vi "Jeremy Example.vi"() -> ()   [LabVIEW 2016]
panel:
  in  "Path":path
  out "Waveform Graph 2":dbl[](graph)
  out "Time Stamp":timestamp
  out "Waveform Graph":dbl[](graph)
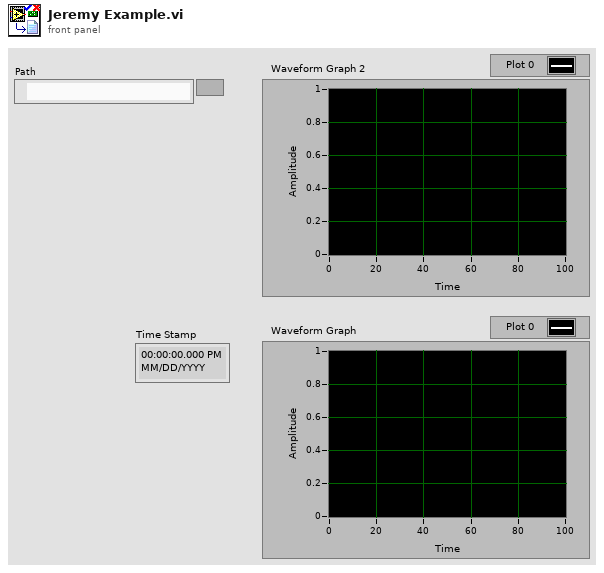
[diagram p1: front panel]
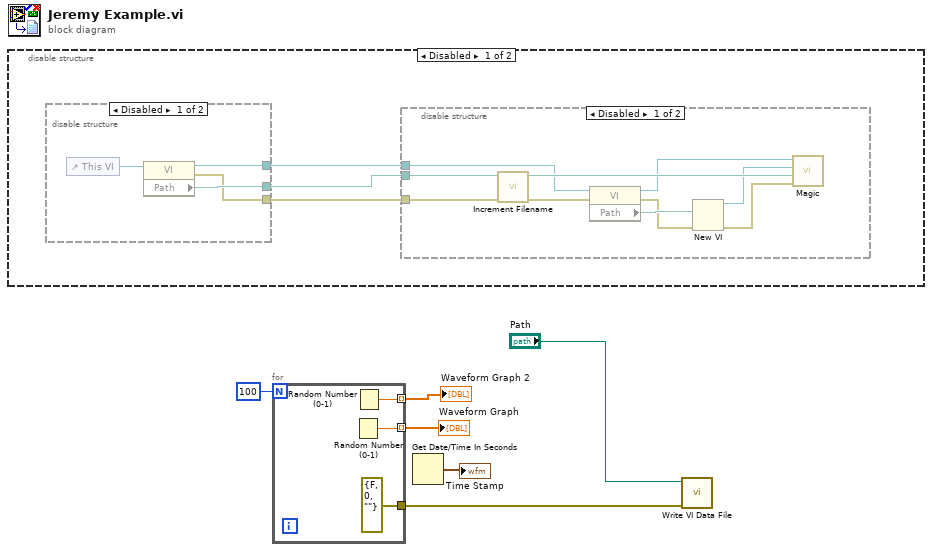
[diagram p0: block diagram]
diagram:
  n1 = disable-structure shown="Disabled" {
    frame Disabled {
      n2 = disable-structure shown="Disabled" {
        disable-tunnel: [w22 _] -> w9
        disable-tunnel: [w21 _] -> w8
        disable-tunnel: [w20 _] -> w7
        frame Disabled {
          n3 = control-ref of="This VI"() -> (w23:refnum<vi>)
          n4 = property class="VI"(reference=w23) -> (reference out=w21:refnum<vi>, error out=w20:errorcluster, "Path"=w22:path)  [unwired: 1 in]
        }
        frame Enabled {
        }
      }
      n5 = disable-structure shown="Disabled" {
        disable-tunnel: w9 -> [w19 _]
        disable-tunnel: w7 -> [w17 _]
        disable-tunnel: w8 -> [w11 _]
        frame Disabled {
          n6 = call <userlib>:"Increment Filename.vi"("error in (no error)"=w17, "Path"=w19) -> ("error out"=w12:errorcluster, "Modified Path"=w18:path)  [unwired: 8 in]
          n7 = property class="VI"(reference=w11, error in=w12) -> (reference out=w10:refnum<vi>, error out=w14:errorcluster, "Path"=w16:path)
          n8 = New VI(8:w14, 10:w16) -> (0:w15:errorcluster, 3:w13:refnum<vi>)  [unwired: 5 in]
          n9 = call "Magic.vi"("error in"=w15, "Target Path"=w18, "Target reference"=w13, "Parent ref"=w10) -> ()  [unwired: 7 in, 1 out]
        }
        frame Enabled {
        }
      }
    }
    frame Enabled {
    }
  }
  n10 = for {
    N: 100 -> [_]
    tunnel: [w26] -> w5 mode=indexing
    tunnel: [w25] -> w3 mode=indexing
    tunnel: [errorcluster {"status"=FALSE, "code"=0, "source"=""} ("error in")] -> w2
    n11 = Random Number (0-1)() -> (number: 0 to 1=w26:dbl)
    n12 = Random Number (0-1)() -> (number: 0 to 1=w25:dbl)
  }
  "Waveform Graph" <- w5
  "Waveform Graph 2" <- w3
  n13 = Get Date/Time In Seconds() -> (seconds since 1Jan1904=→"Time Stamp":timestamp)
  n14 = call "Write VI Data File.vi"("error in"=w2, "Path"="Path") -> ()  [unwired: 8 in, 2 out]
